vi "MoveLift.vi"(11 "Arm is Up?":bool) -> (3 "Updated Bool":bool)   [LabVIEW 2016, in "LEGO-PMR.lvrbt"]
uses:
  LEGO-PMR.lvrbt
  <vilib>/NXT/Block Support/NXT_OutputPort.ctl
  <vilib>/NXT/NXTIO Xnodes/NXTIONodeSubVIs/NXTMotorRunDistance.vi
  <vilib>/NXT/NXTIO Xnodes/AddressXNode/NXTIOAddress.xnode
  <vilib>/NXT/Subs/LVHSConnector.ctl
  <vilib>/NXT/NXTIO Xnodes/NXTIOXNode/NXTIO.xnode
  <vilib>/NXT/LegoClasses/BrickReference/BrickReference.lvclass
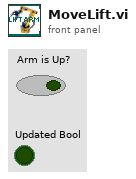
[diagram p1: front panel]
types:
  T1 = typedef "NXT_OutputPort.ctl" = u8
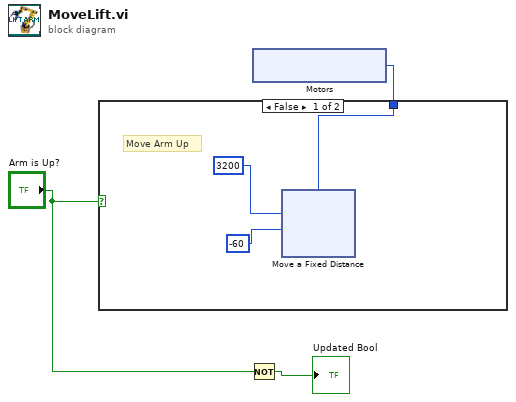
[diagram p0: block diagram]
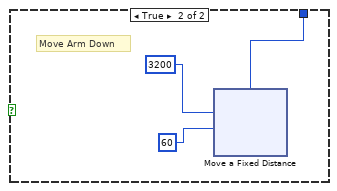
[diagram p2: hidden frame]
diagram:
  n1 = Not(x="Arm is Up?") -> (.not. x?=→"Updated Bool":bool)
  n2 = xnode "Motors"() -> ("Motor"=w3:T1)
  n3 = case shown="False" "Arm is Up?" {
    tunnel: w3 -> [w4 w17]
    frame False {
      # "Move Arm Up"
      n4 = xnode "Move a Fixed Distance"("Speed 1"=-60, "Distance 1"=3200, "Motors"=w4) -> ()  [unwired: 1 in, 1 out]
    }
    frame True {
      # "Move Arm Down"
      n5 = xnode "Move a Fixed Distance"("Speed 1"=60, "Distance 1"=3200, "Motors"=w17) -> ()  [unwired: 1 in, 1 out]
    }
  }
